vi "The Imperial March.vi"(10 "NXT In":T1) -> (2 "NXT Out":T1)   [LabVIEW 2015, in "Katequil.lvrbt"]
uses:
  Katequil/Katequil.lvrbt
  <vilib>/NXT/Subs/LVHSConnector.ctl
  <vilib>/NXT/LegoClasses/BrickReference/BrickReference.lvclass
  <vilib>/NXT/Dual Mode Library/Sound/Tone.vi
  <vilib>/NXT/Dual Mode Library/Waits/Wait_Num(msec).vi
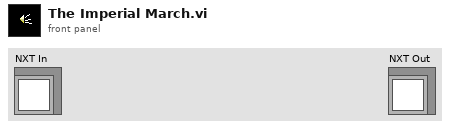
[diagram p1: front panel]
types:
  T1 = typedef "LVHSConnector.ctl" = refnum<class "BrickReference.lvclass">
diagram:
  n1 = call-poly <vilib>:"PolySound.vi"("Duration (500 ms)"=u16 51, "NXT/EV3"="NXT In", "Tone (440 Hz)"=u16 587) -> ("NXT/EV3"=w388:T1)  [unwired: 1 in]
  n2 = call-poly <vilib>:"PolyWait.vi"("Time (100 msec)"=u32 563, "NXT/EV3"=w388) -> ("NXT/EV3"=w383:T1)  [unwired: 2 in]
  n3 = call-poly <vilib>:"PolySound.vi"("Duration (500 ms)"=u16 51, "NXT/EV3"=w383, "Tone (440 Hz)"=u16 587) -> ("NXT/EV3"=w384:T1)  [unwired: 1 in]
  n4 = call-poly <vilib>:"PolyWait.vi"("Time (100 msec)"=u32 563, "NXT/EV3"=w384) -> ("NXT/EV3"=w378:T1)  [unwired: 2 in]
  n5 = call-poly <vilib>:"PolySound.vi"("Duration (500 ms)"=u16 51, "NXT/EV3"=w378, "Tone (440 Hz)"=u16 587) -> ("NXT/EV3"=w379:T1)  [unwired: 1 in]
  n6 = call-poly <vilib>:"PolyWait.vi"("Time (100 msec)"=u32 563, "NXT/EV3"=w379) -> ("NXT/EV3"=w373:T1)  [unwired: 2 in]
  n7 = call-poly <vilib>:"PolySound.vi"("Duration (500 ms)"=u16 34, "NXT/EV3"=w373, "Tone (440 Hz)"=u16 466) -> ("NXT/EV3"=w374:T1)  [unwired: 1 in]
  n8 = call-poly <vilib>:"PolyWait.vi"("Time (100 msec)"=u32 375, "NXT/EV3"=w374) -> ("NXT/EV3"=w368:T1)  [unwired: 2 in]
  n9 = call-poly <vilib>:"PolySound.vi"("Duration (500 ms)"=u16 17, "NXT/EV3"=w368, "Tone (440 Hz)"=u16 698) -> ("NXT/EV3"=w369:T1)  [unwired: 1 in]
  n10 = call-poly <vilib>:"PolyWait.vi"("Time (100 msec)"=u32 188, "NXT/EV3"=w369) -> ("NXT/EV3"=w363:T1)  [unwired: 2 in]
  n11 = call-poly <vilib>:"PolySound.vi"("Duration (500 ms)"=u16 51, "NXT/EV3"=w363, "Tone (440 Hz)"=u16 587) -> ("NXT/EV3"=w364:T1)  [unwired: 1 in]
  n12 = call-poly <vilib>:"PolyWait.vi"("Time (100 msec)"=u32 563, "NXT/EV3"=w364) -> ("NXT/EV3"=w358:T1)  [unwired: 2 in]
  n13 = call-poly <vilib>:"PolySound.vi"("Duration (500 ms)"=u16 34, "NXT/EV3"=w358, "Tone (440 Hz)"=u16 466) -> ("NXT/EV3"=w359:T1)  [unwired: 1 in]
  n14 = call-poly <vilib>:"PolyWait.vi"("Time (100 msec)"=u32 375, "NXT/EV3"=w359) -> ("NXT/EV3"=w353:T1)  [unwired: 2 in]
  n15 = call-poly <vilib>:"PolySound.vi"("Duration (500 ms)"=u16 17, "NXT/EV3"=w353, "Tone (440 Hz)"=u16 698) -> ("NXT/EV3"=w354:T1)  [unwired: 1 in]
  n16 = call-poly <vilib>:"PolyWait.vi"("Time (100 msec)"=u32 188, "NXT/EV3"=w354) -> ("NXT/EV3"=w348:T1)  [unwired: 2 in]
  n17 = call-poly <vilib>:"PolySound.vi"("Duration (500 ms)"=u16 101, "NXT/EV3"=w348, "Tone (440 Hz)"=u16 587) -> ("NXT/EV3"=w349:T1)  [unwired: 1 in]
  n18 = call-poly <vilib>:"PolyWait.vi"("Time (100 msec)"=u32 112, "NXT/EV3"=w349) -> ("NXT/EV3"=w343:T1)  [unwired: 2 in]
  n19 = call-poly <vilib>:"PolySound.vi"("Duration (500 ms)"=u16 8, "NXT/EV3"=w343, "Tone (440 Hz)"=u16 0) -> ("NXT/EV3"=w344:T1)  [unwired: 1 in]
  n20 = call-poly <vilib>:"PolyWait.vi"("Time (100 msec)"=u32 94, "NXT/EV3"=w344) -> ("NXT/EV3"=w338:T1)  [unwired: 2 in]
  n21 = call-poly <vilib>:"PolySound.vi"("Duration (500 ms)"=u16 51, "NXT/EV3"=w338, "Tone (440 Hz)"=u16 880) -> ("NXT/EV3"=w339:T1)  [unwired: 1 in]
  n22 = call-poly <vilib>:"PolyWait.vi"("Time (100 msec)"=u32 563, "NXT/EV3"=w339) -> ("NXT/EV3"=w333:T1)  [unwired: 2 in]
  n23 = call-poly <vilib>:"PolySound.vi"("Duration (500 ms)"=u16 51, "NXT/EV3"=w333, "Tone (440 Hz)"=u16 880) -> ("NXT/EV3"=w334:T1)  [unwired: 1 in]
  n24 = call-poly <vilib>:"PolyWait.vi"("Time (100 msec)"=u32 563, "NXT/EV3"=w334) -> ("NXT/EV3"=w328:T1)  [unwired: 2 in]
  n25 = call-poly <vilib>:"PolySound.vi"("Duration (500 ms)"=u16 51, "NXT/EV3"=w328, "Tone (440 Hz)"=u16 880) -> ("NXT/EV3"=w329:T1)  [unwired: 1 in]
  n26 = call-poly <vilib>:"PolyWait.vi"("Time (100 msec)"=u32 563, "NXT/EV3"=w329) -> ("NXT/EV3"=w323:T1)  [unwired: 2 in]
  n27 = call-poly <vilib>:"PolySound.vi"("Duration (500 ms)"=u16 34, "NXT/EV3"=w323, "Tone (440 Hz)"=u16 932) -> ("NXT/EV3"=w324:T1)  [unwired: 1 in]
  n28 = call-poly <vilib>:"PolyWait.vi"("Time (100 msec)"=u32 375, "NXT/EV3"=w324) -> ("NXT/EV3"=w318:T1)  [unwired: 2 in]
  n29 = call-poly <vilib>:"PolySound.vi"("Duration (500 ms)"=u16 17, "NXT/EV3"=w318, "Tone (440 Hz)"=u16 698) -> ("NXT/EV3"=w319:T1)  [unwired: 1 in]
  n30 = call-poly <vilib>:"PolyWait.vi"("Time (100 msec)"=u32 188, "NXT/EV3"=w319) -> ("NXT/EV3"=w313:T1)  [unwired: 2 in]
  n31 = call-poly <vilib>:"PolySound.vi"("Duration (500 ms)"=u16 51, "NXT/EV3"=w313, "Tone (440 Hz)"=u16 554) -> ("NXT/EV3"=w314:T1)  [unwired: 1 in]
  n32 = call-poly <vilib>:"PolyWait.vi"("Time (100 msec)"=u32 563, "NXT/EV3"=w314) -> ("NXT/EV3"=w308:T1)  [unwired: 2 in]
  n33 = call-poly <vilib>:"PolySound.vi"("Duration (500 ms)"=u16 34, "NXT/EV3"=w308, "Tone (440 Hz)"=u16 466) -> ("NXT/EV3"=w309:T1)  [unwired: 1 in]
  n34 = call-poly <vilib>:"PolyWait.vi"("Time (100 msec)"=u32 375, "NXT/EV3"=w309) -> ("NXT/EV3"=w304:T1)  [unwired: 2 in]
  n35 = call-poly <vilib>:"PolySound.vi"("Duration (500 ms)"=u16 17, "NXT/EV3"=w304, "Tone (440 Hz)"=u16 698) -> ("NXT/EV3"=w305:T1)  [unwired: 1 in]
  n36 = call-poly <vilib>:"PolyWait.vi"("Time (100 msec)"=u32 188, "NXT/EV3"=w305) -> ("NXT/EV3"=w298:T1)  [unwired: 2 in]
  n37 = call-poly <vilib>:"PolySound.vi"("Duration (500 ms)"=u16 101, "NXT/EV3"=w298, "Tone (440 Hz)"=u16 587) -> ("NXT/EV3"=w299:T1)  [unwired: 1 in]
  n38 = call-poly <vilib>:"PolyWait.vi"("Time (100 msec)"=u32 1125, "NXT/EV3"=w299) -> ("NXT/EV3"=w293:T1)  [unwired: 2 in]
  n39 = call-poly <vilib>:"PolySound.vi"("Duration (500 ms)"=u16 8, "NXT/EV3"=w293, "Tone (440 Hz)"=u16 0) -> ("NXT/EV3"=w294:T1)  [unwired: 1 in]
  n40 = call-poly <vilib>:"PolyWait.vi"("Time (100 msec)"=u32 94, "NXT/EV3"=w294) -> ("NXT/EV3"=w288:T1)  [unwired: 2 in]
  n41 = call-poly <vilib>:"PolySound.vi"("Duration (500 ms)"=u16 51, "NXT/EV3"=w288, "Tone (440 Hz)"=u16 880) -> ("NXT/EV3"=w289:T1)  [unwired: 1 in]
  n42 = call-poly <vilib>:"PolyWait.vi"("Time (100 msec)"=u32 563, "NXT/EV3"=w289) -> ("NXT/EV3"=w283:T1)  [unwired: 2 in]
  n43 = call-poly <vilib>:"PolySound.vi"("Duration (500 ms)"=u16 51, "NXT/EV3"=w283, "Tone (440 Hz)"=u16 587) -> ("NXT/EV3"=w284:T1)  [unwired: 1 in]
  n44 = call-poly <vilib>:"PolyWait.vi"("Time (100 msec)"=u32 563, "NXT/EV3"=w284) -> ("NXT/EV3"=w278:T1)  [unwired: 2 in]
  n45 = call-poly <vilib>:"PolySound.vi"("Duration (500 ms)"=u16 34, "NXT/EV3"=w278, "Tone (440 Hz)"=u16 587) -> ("NXT/EV3"=w279:T1)  [unwired: 1 in]
  n46 = call-poly <vilib>:"PolyWait.vi"("Time (100 msec)"=u32 375, "NXT/EV3"=w279) -> ("NXT/EV3"=w273:T1)  [unwired: 2 in]
  n47 = call-poly <vilib>:"PolySound.vi"("Duration (500 ms)"=u16 17, "NXT/EV3"=w273, "Tone (440 Hz)"=u16 587) -> ("NXT/EV3"=w274:T1)  [unwired: 1 in]
  n48 = call-poly <vilib>:"PolyWait.vi"("Time (100 msec)"=u32 188, "NXT/EV3"=w274) -> ("NXT/EV3"=w268:T1)  [unwired: 2 in]
  n49 = call-poly <vilib>:"PolySound.vi"("Duration (500 ms)"=u16 34, "NXT/EV3"=w268, "Tone (440 Hz)"=u16 880) -> ("NXT/EV3"=w269:T1)  [unwired: 1 in]
  n50 = call-poly <vilib>:"PolyWait.vi"("Time (100 msec)"=u32 375, "NXT/EV3"=w269) -> ("NXT/EV3"=w263:T1)  [unwired: 2 in]
  n51 = call-poly <vilib>:"PolySound.vi"("Duration (500 ms)"=u16 8, "NXT/EV3"=w263, "Tone (440 Hz)"=u16 0) -> ("NXT/EV3"=w264:T1)  [unwired: 1 in]
  n52 = call-poly <vilib>:"PolyWait.vi"("Time (100 msec)"=u32 94, "NXT/EV3"=w264) -> ("NXT/EV3"=w258:T1)  [unwired: 2 in]
  n53 = call-poly <vilib>:"PolySound.vi"("Duration (500 ms)"=u16 34, "NXT/EV3"=w258, "Tone (440 Hz)"=u16 831) -> ("NXT/EV3"=w259:T1)  [unwired: 1 in]
  n54 = call-poly <vilib>:"PolyWait.vi"("Time (100 msec)"=u32 375, "NXT/EV3"=w259) -> ("NXT/EV3"=w253:T1)  [unwired: 2 in]
  n55 = call-poly <vilib>:"PolySound.vi"("Duration (500 ms)"=u16 17, "NXT/EV3"=w253, "Tone (440 Hz)"=u16 784) -> ("NXT/EV3"=w254:T1)  [unwired: 1 in]
  n56 = call-poly <vilib>:"PolyWait.vi"("Time (100 msec)"=u32 188, "NXT/EV3"=w254) -> ("NXT/EV3"=w248:T1)  [unwired: 2 in]
  n57 = call-poly <vilib>:"PolySound.vi"("Duration (500 ms)"=u16 17, "NXT/EV3"=w248, "Tone (440 Hz)"=u16 987) -> ("NXT/EV3"=w249:T1)  [unwired: 1 in]
  n58 = call-poly <vilib>:"PolyWait.vi"("Time (100 msec)"=u32 188, "NXT/EV3"=w249) -> ("NXT/EV3"=w243:T1)  [unwired: 2 in]
  n59 = call-poly <vilib>:"PolySound.vi"("Duration (500 ms)"=u16 17, "NXT/EV3"=w243, "Tone (440 Hz)"=u16 932) -> ("NXT/EV3"=w244:T1)  [unwired: 1 in]
  n60 = call-poly <vilib>:"PolyWait.vi"("Time (100 msec)"=u32 188, "NXT/EV3"=w244) -> ("NXT/EV3"=w238:T1)  [unwired: 2 in]
  n61 = call-poly <vilib>:"PolySound.vi"("Duration (500 ms)"=u16 17, "NXT/EV3"=w238, "Tone (440 Hz)"=u16 932) -> ("NXT/EV3"=w239:T1)  [unwired: 1 in]
  n62 = call-poly <vilib>:"PolyWait.vi"("Time (100 msec)"=u32 188, "NXT/EV3"=w239) -> ("NXT/EV3"=w233:T1)  [unwired: 2 in]
  n63 = call-poly <vilib>:"PolySound.vi"("Duration (500 ms)"=u16 34, "NXT/EV3"=w233, "Tone (440 Hz)"=u16 987) -> ("NXT/EV3"=w234:T1)  [unwired: 1 in]
  n64 = call-poly <vilib>:"PolyWait.vi"("Time (100 msec)"=u32 375, "NXT/EV3"=w234) -> ("NXT/EV3"=w228:T1)  [unwired: 2 in]
  n65 = call-poly <vilib>:"PolySound.vi"("Duration (500 ms)"=u16 8, "NXT/EV3"=w228, "Tone (440 Hz)"=u16 0) -> ("NXT/EV3"=w229:T1)  [unwired: 1 in]
  n66 = call-poly <vilib>:"PolyWait.vi"("Time (100 msec)"=u32 94, "NXT/EV3"=w229) -> ("NXT/EV3"=w223:T1)  [unwired: 2 in]
  n67 = call-poly <vilib>:"PolySound.vi"("Duration (500 ms)"=u16 34, "NXT/EV3"=w223, "Tone (440 Hz)"=u16 783) -> ("NXT/EV3"=w224:T1)  [unwired: 1 in]
  n68 = call-poly <vilib>:"PolyWait.vi"("Time (100 msec)"=u32 375, "NXT/EV3"=w224) -> ("NXT/EV3"=w218:T1)  [unwired: 2 in]
  n69 = call-poly <vilib>:"PolySound.vi"("Duration (500 ms)"=u16 17, "NXT/EV3"=w218, "Tone (440 Hz)"=u16 739) -> ("NXT/EV3"=w219:T1)  [unwired: 1 in]
  n70 = call-poly <vilib>:"PolyWait.vi"("Time (100 msec)"=u32 188, "NXT/EV3"=w219) -> ("NXT/EV3"=w213:T1)  [unwired: 2 in]
  n71 = call-poly <vilib>:"PolySound.vi"("Duration (500 ms)"=u16 17, "NXT/EV3"=w213, "Tone (440 Hz)"=u16 698) -> ("NXT/EV3"=w214:T1)  [unwired: 1 in]
  n72 = call-poly <vilib>:"PolyWait.vi"("Time (100 msec)"=u32 188, "NXT/EV3"=w214) -> ("NXT/EV3"=w208:T1)  [unwired: 2 in]
  n73 = call-poly <vilib>:"PolySound.vi"("Duration (500 ms)"=u16 17, "NXT/EV3"=w208, "Tone (440 Hz)"=u16 659) -> ("NXT/EV3"=w209:T1)  [unwired: 1 in]
  n74 = call-poly <vilib>:"PolyWait.vi"("Time (100 msec)"=u32 188, "NXT/EV3"=w209) -> ("NXT/EV3"=w203:T1)  [unwired: 2 in]
  n75 = call-poly <vilib>:"PolySound.vi"("Duration (500 ms)"=u16 34, "NXT/EV3"=w203, "Tone (440 Hz)"=u16 698) -> ("NXT/EV3"=w204:T1)  [unwired: 1 in]
  n76 = call-poly <vilib>:"PolyWait.vi"("Time (100 msec)"=u32 375, "NXT/EV3"=w204) -> ("NXT/EV3"=w198:T1)  [unwired: 2 in]
  n77 = call-poly <vilib>:"PolySound.vi"("Duration (500 ms)"=u16 8, "NXT/EV3"=w198, "Tone (440 Hz)"=u16 0) -> ("NXT/EV3"=w199:T1)  [unwired: 1 in]
  n78 = call-poly <vilib>:"PolyWait.vi"("Time (100 msec)"=u32 94, "NXT/EV3"=w199) -> ("NXT/EV3"=w193:T1)  [unwired: 2 in]
  n79 = call-poly <vilib>:"PolySound.vi"("Duration (500 ms)"=u16 17, "NXT/EV3"=w193, "Tone (440 Hz)"=u16 466) -> ("NXT/EV3"=w194:T1)  [unwired: 1 in]
  n80 = call-poly <vilib>:"PolyWait.vi"("Time (100 msec)"=u32 188, "NXT/EV3"=w194) -> ("NXT/EV3"=w188:T1)  [unwired: 2 in]
  n81 = call-poly <vilib>:"PolySound.vi"("Duration (500 ms)"=u16 34, "NXT/EV3"=w188, "Tone (440 Hz)"=u16 554) -> ("NXT/EV3"=w189:T1)  [unwired: 1 in]
  n82 = call-poly <vilib>:"PolyWait.vi"("Time (100 msec)"=u32 375, "NXT/EV3"=w189) -> ("NXT/EV3"=w183:T1)  [unwired: 2 in]
  n83 = call-poly <vilib>:"PolySound.vi"("Duration (500 ms)"=u16 8, "NXT/EV3"=w183, "Tone (440 Hz)"=u16 0) -> ("NXT/EV3"=w184:T1)  [unwired: 1 in]
  n84 = call-poly <vilib>:"PolyWait.vi"("Time (100 msec)"=u32 94, "NXT/EV3"=w184) -> ("NXT/EV3"=w178:T1)  [unwired: 2 in]
  n85 = call-poly <vilib>:"PolySound.vi"("Duration (500 ms)"=u16 34, "NXT/EV3"=w178, "Tone (440 Hz)"=u16 466) -> ("NXT/EV3"=w179:T1)  [unwired: 1 in]
  n86 = call-poly <vilib>:"PolyWait.vi"("Time (100 msec)"=u32 375, "NXT/EV3"=w179) -> ("NXT/EV3"=w172:T1)  [unwired: 2 in]
  n87 = call-poly <vilib>:"PolySound.vi"("Duration (500 ms)"=u16 17, "NXT/EV3"=w172, "Tone (440 Hz)"=u16 554) -> ("NXT/EV3"=w173:T1)  [unwired: 1 in]
  n88 = call-poly <vilib>:"PolyWait.vi"("Time (100 msec)"=u32 188, "NXT/EV3"=w173) -> ("NXT/EV3"=w167:T1)  [unwired: 2 in]
  n89 = call-poly <vilib>:"PolySound.vi"("Duration (500 ms)"=u16 51, "NXT/EV3"=w167, "Tone (440 Hz)"=u16 698) -> ("NXT/EV3"=w168:T1)  [unwired: 1 in]
  n90 = call-poly <vilib>:"PolyWait.vi"("Time (100 msec)"=u32 563, "NXT/EV3"=w168) -> ("NXT/EV3"=w162:T1)  [unwired: 2 in]
  n91 = call-poly <vilib>:"PolySound.vi"("Duration (500 ms)"=u16 34, "NXT/EV3"=w162, "Tone (440 Hz)"=u16 587) -> ("NXT/EV3"=w163:T1)  [unwired: 1 in]
  n92 = call-poly <vilib>:"PolyWait.vi"("Time (100 msec)"=u32 375, "NXT/EV3"=w163) -> ("NXT/EV3"=w157:T1)  [unwired: 2 in]
  n93 = call-poly <vilib>:"PolySound.vi"("Duration (500 ms)"=u16 17, "NXT/EV3"=w157, "Tone (440 Hz)"=u16 698) -> ("NXT/EV3"=w158:T1)  [unwired: 1 in]
  n94 = call-poly <vilib>:"PolyWait.vi"("Time (100 msec)"=u32 188, "NXT/EV3"=w158) -> ("NXT/EV3"=w152:T1)  [unwired: 2 in]
  n95 = call-poly <vilib>:"PolySound.vi"("Duration (500 ms)"=u16 101, "NXT/EV3"=w152, "Tone (440 Hz)"=u16 880) -> ("NXT/EV3"=w153:T1)  [unwired: 1 in]
  n96 = call-poly <vilib>:"PolyWait.vi"("Time (100 msec)"=u32 1125, "NXT/EV3"=w153) -> ("NXT/EV3"=w147:T1)  [unwired: 2 in]
  n97 = call-poly <vilib>:"PolySound.vi"("Duration (500 ms)"=u16 8, "NXT/EV3"=w147, "Tone (440 Hz)"=u16 0) -> ("NXT/EV3"=w148:T1)  [unwired: 1 in]
  n98 = call-poly <vilib>:"PolyWait.vi"("Time (100 msec)"=u32 94, "NXT/EV3"=w148) -> ("NXT/EV3"=w142:T1)  [unwired: 2 in]
  n99 = call-poly <vilib>:"PolySound.vi"("Duration (500 ms)"=u16 51, "NXT/EV3"=w142, "Tone (440 Hz)"=u16 880) -> ("NXT/EV3"=w143:T1)  [unwired: 1 in]
  n100 = call-poly <vilib>:"PolyWait.vi"("Time (100 msec)"=u32 563, "NXT/EV3"=w143) -> ("NXT/EV3"=w137:T1)  [unwired: 2 in]
  n101 = call-poly <vilib>:"PolySound.vi"("Duration (500 ms)"=u16 34, "NXT/EV3"=w137, "Tone (440 Hz)"=u16 587) -> ("NXT/EV3"=w138:T1)  [unwired: 1 in]
  n102 = call-poly <vilib>:"PolyWait.vi"("Time (100 msec)"=u32 375, "NXT/EV3"=w138) -> ("NXT/EV3"=w132:T1)  [unwired: 2 in]
  n103 = call-poly <vilib>:"PolySound.vi"("Duration (500 ms)"=u16 17, "NXT/EV3"=w132, "Tone (440 Hz)"=u16 587) -> ("NXT/EV3"=w133:T1)  [unwired: 1 in]
  n104 = call-poly <vilib>:"PolyWait.vi"("Time (100 msec)"=u32 188, "NXT/EV3"=w133) -> ("NXT/EV3"=w127:T1)  [unwired: 2 in]
  n105 = call-poly <vilib>:"PolySound.vi"("Duration (500 ms)"=u16 34, "NXT/EV3"=w127, "Tone (440 Hz)"=u16 880) -> ("NXT/EV3"=w128:T1)  [unwired: 1 in]
  n106 = call-poly <vilib>:"PolyWait.vi"("Time (100 msec)"=u32 375, "NXT/EV3"=w128) -> ("NXT/EV3"=w122:T1)  [unwired: 2 in]
  n107 = call-poly <vilib>:"PolySound.vi"("Duration (500 ms)"=u16 8, "NXT/EV3"=w122, "Tone (440 Hz)"=u16 0) -> ("NXT/EV3"=w123:T1)  [unwired: 1 in]
  n108 = call-poly <vilib>:"PolyWait.vi"("Time (100 msec)"=u32 94, "NXT/EV3"=w123) -> ("NXT/EV3"=w117:T1)  [unwired: 2 in]
  n109 = call-poly <vilib>:"PolySound.vi"("Duration (500 ms)"=u16 34, "NXT/EV3"=w117, "Tone (440 Hz)"=u16 831) -> ("NXT/EV3"=w118:T1)  [unwired: 1 in]
  n110 = call-poly <vilib>:"PolyWait.vi"("Time (100 msec)"=u32 375, "NXT/EV3"=w118) -> ("NXT/EV3"=w112:T1)  [unwired: 2 in]
  n111 = call-poly <vilib>:"PolySound.vi"("Duration (500 ms)"=u16 17, "NXT/EV3"=w112, "Tone (440 Hz)"=u16 784) -> ("NXT/EV3"=w113:T1)  [unwired: 1 in]
  n112 = call-poly <vilib>:"PolyWait.vi"("Time (100 msec)"=u32 188, "NXT/EV3"=w113) -> ("NXT/EV3"=w107:T1)  [unwired: 2 in]
  n113 = call-poly <vilib>:"PolySound.vi"("Duration (500 ms)"=u16 17, "NXT/EV3"=w107, "Tone (440 Hz)"=u16 987) -> ("NXT/EV3"=w108:T1)  [unwired: 1 in]
  n114 = call-poly <vilib>:"PolyWait.vi"("Time (100 msec)"=u32 188, "NXT/EV3"=w108) -> ("NXT/EV3"=w102:T1)  [unwired: 2 in]
  n115 = call-poly <vilib>:"PolySound.vi"("Duration (500 ms)"=u16 17, "NXT/EV3"=w102, "Tone (440 Hz)"=u16 932) -> ("NXT/EV3"=w103:T1)  [unwired: 1 in]
  n116 = call-poly <vilib>:"PolyWait.vi"("Time (100 msec)"=u32 188, "NXT/EV3"=w103) -> ("NXT/EV3"=w97:T1)  [unwired: 2 in]
  n117 = call-poly <vilib>:"PolySound.vi"("Duration (500 ms)"=u16 34, "NXT/EV3"=w97, "Tone (440 Hz)"=u16 987) -> ("NXT/EV3"=w98:T1)  [unwired: 1 in]
  n118 = call-poly <vilib>:"PolyWait.vi"("Time (100 msec)"=u32 375, "NXT/EV3"=w98) -> ("NXT/EV3"=w92:T1)  [unwired: 2 in]
  n119 = call-poly <vilib>:"PolySound.vi"("Duration (500 ms)"=u16 8, "NXT/EV3"=w92, "Tone (440 Hz)"=u16 0) -> ("NXT/EV3"=w93:T1)  [unwired: 1 in]
  n120 = call-poly <vilib>:"PolyWait.vi"("Time (100 msec)"=u32 94, "NXT/EV3"=w93) -> ("NXT/EV3"=w87:T1)  [unwired: 2 in]
  n121 = call-poly <vilib>:"PolySound.vi"("Duration (500 ms)"=u16 17, "NXT/EV3"=w87, "Tone (440 Hz)"=u16 622) -> ("NXT/EV3"=w88:T1)  [unwired: 1 in]
  n122 = call-poly <vilib>:"PolyWait.vi"("Time (100 msec)"=u32 188, "NXT/EV3"=w88) -> ("NXT/EV3"=w82:T1)  [unwired: 2 in]
  n123 = call-poly <vilib>:"PolySound.vi"("Duration (500 ms)"=u16 34, "NXT/EV3"=w82, "Tone (440 Hz)"=u16 830) -> ("NXT/EV3"=w83:T1)  [unwired: 1 in]
  n124 = call-poly <vilib>:"PolyWait.vi"("Time (100 msec)"=u32 375, "NXT/EV3"=w83) -> ("NXT/EV3"=w77:T1)  [unwired: 2 in]
  n125 = call-poly <vilib>:"PolySound.vi"("Duration (500 ms)"=u16 8, "NXT/EV3"=w77, "Tone (440 Hz)"=u16 0) -> ("NXT/EV3"=w78:T1)  [unwired: 1 in]
  n126 = call-poly <vilib>:"PolyWait.vi"("Time (100 msec)"=u32 94, "NXT/EV3"=w78) -> ("NXT/EV3"=w72:T1)  [unwired: 2 in]
  n127 = call-poly <vilib>:"PolySound.vi"("Duration (500 ms)"=u16 34, "NXT/EV3"=w72, "Tone (440 Hz)"=u16 783) -> ("NXT/EV3"=w73:T1)  [unwired: 1 in]
  n128 = call-poly <vilib>:"PolyWait.vi"("Time (100 msec)"=u32 375, "NXT/EV3"=w73) -> ("NXT/EV3"=w67:T1)  [unwired: 2 in]
  n129 = call-poly <vilib>:"PolySound.vi"("Duration (500 ms)"=u16 17, "NXT/EV3"=w67, "Tone (440 Hz)"=u16 739) -> ("NXT/EV3"=w68:T1)  [unwired: 1 in]
  n130 = call-poly <vilib>:"PolyWait.vi"("Time (100 msec)"=u32 188, "NXT/EV3"=w68) -> ("NXT/EV3"=w62:T1)  [unwired: 2 in]
  n131 = call-poly <vilib>:"PolySound.vi"("Duration (500 ms)"=u16 17, "NXT/EV3"=w62, "Tone (440 Hz)"=u16 698) -> ("NXT/EV3"=w63:T1)  [unwired: 1 in]
  n132 = call-poly <vilib>:"PolyWait.vi"("Time (100 msec)"=u32 188, "NXT/EV3"=w63) -> ("NXT/EV3"=w57:T1)  [unwired: 2 in]
  n133 = call-poly <vilib>:"PolySound.vi"("Duration (500 ms)"=u16 17, "NXT/EV3"=w57, "Tone (440 Hz)"=u16 659) -> ("NXT/EV3"=w58:T1)  [unwired: 1 in]
  n134 = call-poly <vilib>:"PolyWait.vi"("Time (100 msec)"=u32 188, "NXT/EV3"=w58) -> ("NXT/EV3"=w52:T1)  [unwired: 2 in]
  n135 = call-poly <vilib>:"PolySound.vi"("Duration (500 ms)"=u16 34, "NXT/EV3"=w52, "Tone (440 Hz)"=u16 698) -> ("NXT/EV3"=w53:T1)  [unwired: 1 in]
  n136 = call-poly <vilib>:"PolyWait.vi"("Time (100 msec)"=u32 375, "NXT/EV3"=w53) -> ("NXT/EV3"=w47:T1)  [unwired: 2 in]
  n137 = call-poly <vilib>:"PolySound.vi"("Duration (500 ms)"=u16 8, "NXT/EV3"=w47, "Tone (440 Hz)"=u16 0) -> ("NXT/EV3"=w48:T1)  [unwired: 1 in]
  n138 = call-poly <vilib>:"PolyWait.vi"("Time (100 msec)"=u32 94, "NXT/EV3"=w48) -> ("NXT/EV3"=w42:T1)  [unwired: 2 in]
  n139 = call-poly <vilib>:"PolySound.vi"("Duration (500 ms)"=u16 17, "NXT/EV3"=w42, "Tone (440 Hz)"=u16 466) -> ("NXT/EV3"=w43:T1)  [unwired: 1 in]
  n140 = call-poly <vilib>:"PolyWait.vi"("Time (100 msec)"=u32 188, "NXT/EV3"=w43) -> ("NXT/EV3"=w37:T1)  [unwired: 2 in]
  n141 = call-poly <vilib>:"PolySound.vi"("Duration (500 ms)"=u16 34, "NXT/EV3"=w37, "Tone (440 Hz)"=u16 554) -> ("NXT/EV3"=w38:T1)  [unwired: 1 in]
  n142 = call-poly <vilib>:"PolyWait.vi"("Time (100 msec)"=u32 375, "NXT/EV3"=w38) -> ("NXT/EV3"=w32:T1)  [unwired: 2 in]
  n143 = call-poly <vilib>:"PolySound.vi"("Duration (500 ms)"=u16 8, "NXT/EV3"=w32, "Tone (440 Hz)"=u16 0) -> ("NXT/EV3"=w33:T1)  [unwired: 1 in]
  n144 = call-poly <vilib>:"PolyWait.vi"("Time (100 msec)"=u32 94, "NXT/EV3"=w33) -> ("NXT/EV3"=w27:T1)  [unwired: 2 in]
  n145 = call-poly <vilib>:"PolySound.vi"("Duration (500 ms)"=u16 34, "NXT/EV3"=w27, "Tone (440 Hz)"=u16 466) -> ("NXT/EV3"=w28:T1)  [unwired: 1 in]
  n146 = call-poly <vilib>:"PolyWait.vi"("Time (100 msec)"=u32 375, "NXT/EV3"=w28) -> ("NXT/EV3"=w22:T1)  [unwired: 2 in]
  n147 = call-poly <vilib>:"PolySound.vi"("Duration (500 ms)"=u16 17, "NXT/EV3"=w22, "Tone (440 Hz)"=u16 698) -> ("NXT/EV3"=w23:T1)  [unwired: 1 in]
  n148 = call-poly <vilib>:"PolyWait.vi"("Time (100 msec)"=u32 188, "NXT/EV3"=w23) -> ("NXT/EV3"=w17:T1)  [unwired: 2 in]
  n149 = call-poly <vilib>:"PolySound.vi"("Duration (500 ms)"=u16 51, "NXT/EV3"=w17, "Tone (440 Hz)"=u16 587) -> ("NXT/EV3"=w18:T1)  [unwired: 1 in]
  n150 = call-poly <vilib>:"PolyWait.vi"("Time (100 msec)"=u32 563, "NXT/EV3"=w18) -> ("NXT/EV3"=w12:T1)  [unwired: 2 in]
  n151 = call-poly <vilib>:"PolySound.vi"("Duration (500 ms)"=u16 34, "NXT/EV3"=w12, "Tone (440 Hz)"=u16 466) -> ("NXT/EV3"=w13:T1)  [unwired: 1 in]
  n152 = call-poly <vilib>:"PolyWait.vi"("Time (100 msec)"=u32 375, "NXT/EV3"=w13) -> ("NXT/EV3"=w7:T1)  [unwired: 2 in]
  n153 = call-poly <vilib>:"PolySound.vi"("Duration (500 ms)"=u16 17, "NXT/EV3"=w7, "Tone (440 Hz)"=u16 698) -> ("NXT/EV3"=w8:T1)  [unwired: 1 in]
  n154 = call-poly <vilib>:"PolyWait.vi"("Time (100 msec)"=u32 188, "NXT/EV3"=w8) -> ("NXT/EV3"=w2:T1)  [unwired: 2 in]
  n155 = call-poly <vilib>:"PolySound.vi"("Duration (500 ms)"=u16 101, "NXT/EV3"=w2, "Tone (440 Hz)"=u16 587) -> ("NXT/EV3"=w3:T1)  [unwired: 1 in]
  n156 = call-poly <vilib>:"PolyWait.vi"("Time (100 msec)"=u32 1125, "NXT/EV3"=w3) -> ("NXT/EV3"=→"NXT Out":T1)  [unwired: 2 in]
